vi "Key Reader.vi"(8 "error in":errorcluster, 11 "LTB-1 in":refnum<class "LTB-1.lvclass">) -> (0 "error out":errorcluster, 3 "LTB-1 out":refnum<class "LTB-1.lvclass">)   [LabVIEW 2018, in "LTB-1.lvlib" / "LTB-1.lvclass"]
uses:
  LTB-1.lvclass
  C:/AME Test Engineering/LabVIEW/PPLs/EXFO/Parent/EXFO.lvlibp/EXFO.lvclass
  LTB-1.lvclass/LTB-1.ctl
  PPLs/EXFO/Parent/EXFO.lvlibp/Methods/Read Configuration.vi
  PPLs/Configuration/Configuration.lvlibp/Configuration.lvclass
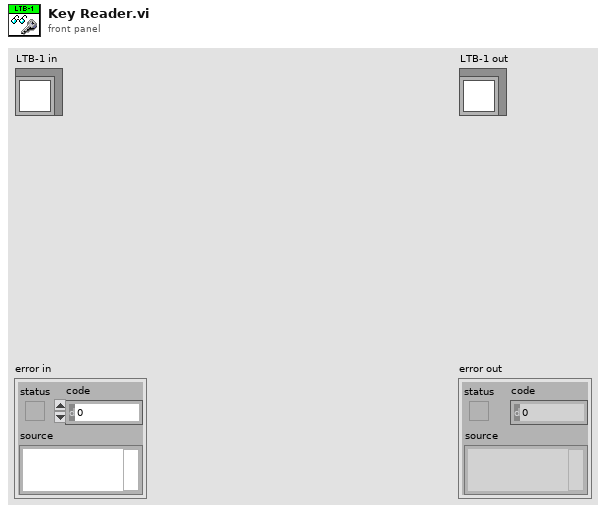
[diagram p1: front panel]
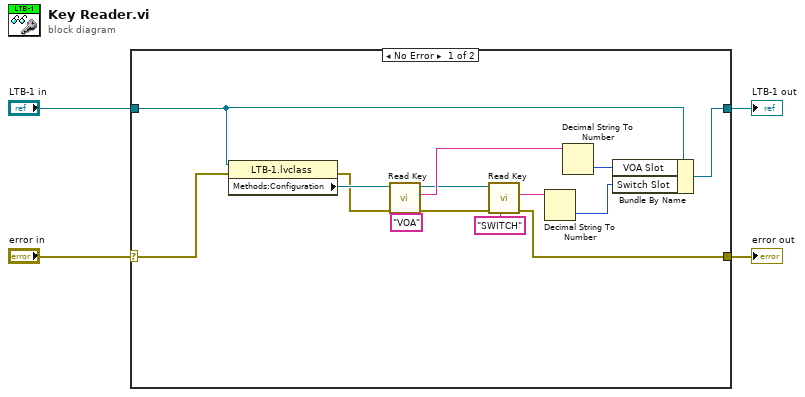
[diagram p0: block diagram]
diagram:
  n1 = case shown="No Error" "error in" {
    selector: "error in" -> [w9 w20]
    tunnel: [w5 w20] -> w3
    tunnel: [w10 w19] -> w1
    tunnel: "LTB-1 in" -> [w13 w19]
    frame No Error {
      n2 = property class="LTB-1.lvclass"(reference=w13, error in=w9) -> (error out=w6:errorcluster, "Methods:Configuration"=w18:refnum<class "Configuration.lvclass">)  [unwired: 1 out]
      n3 = call "Read Key.vi"("Key:"="VOA", "error in"=w6, "Configuration in"=w18) -> ("error out"=w7:errorcluster, "Value"=w15:string, "Configuration out"=w8:refnum<class "Configuration.lvclass">)  [unwired: 6 in]
      n4 = call "Read Key.vi"("Key:"="SWITCH", "error in"=w7, "Configuration in"=w8) -> ("error out"=w5:errorcluster, "Value"=w14:string)  [unwired: 6 in, 1 out]
      n5 = Decimal String To Number(string=w14) -> (number=w11:i32)  [unwired: 2 in, 1 out]
      n6 = Decimal String To Number(string=w15) -> (number=w12:i32)  [unwired: 2 in, 1 out]
      n7 = Bundle By Name(cluster=w13, "VOA Slot"=w12, "Switch Slot"=w11) -> (w10:refnum<class "LTB-1.lvclass">)
    }
    frame Error {
    }
  }
  "error out" <- w3
  "LTB-1 out" <- w1
